vi "metron tester.vi"() -> ()   [LabVIEW 2024]
uses:
  <vilib>/addons/_JKI.lib/REST Client/classes/REST Client/HTTP Header.ctl
  <vilib>/NI/Advanced HTTP Client/Header--Combo Box.ctl
  <vilib>/addons/_JKI.lib/REST Client/classes/REST Client/REST Client.lvclass
  <vilib>/addons/_JKI.lib/Serialization/JSON/JKI JSON Serialization.lvlib
  <vilib>/NI/Advanced HTTP Client/Session.lvclass
panel:
  out "substring":string
  out "Status String":string
  out "text":string
  out "size(s)":i32
  out "Numeric":i32
  out "results":T1(array[cluster])
  out "resulting string":string
  out "Response body":string
  in  "error in (no error)":errorcluster
  out "error out":errorcluster
  in  "resource":string
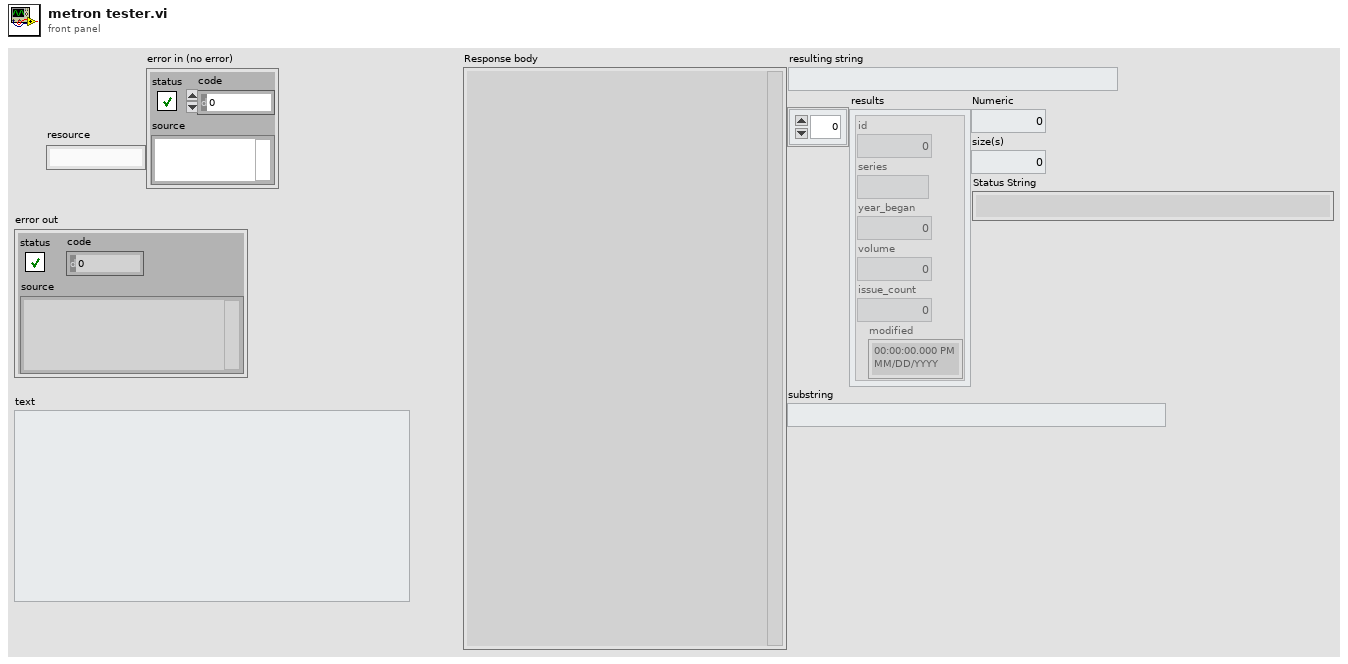
[diagram p1: front panel]
types:
  T1 = cluster{"id":i32, "series":string, "year_began":i32, "volume":i32, "issue_count":i32, "modified":timestamp}[]
  T2 = typedef "REST Client.lvlib/REST Client.lvclass/HTTP Header.ctl" = cluster{"header":T3, "value":string}
  T3 = typedef "lib_NI_Advanced HTTP Client.lvlib/Session.lvclass/Header--Combo Box.ctl" = string
  T4 = cluster{"count":i32, "next":string, "previous":string, "results":cluster{"id":i32, "series":string, "year_began":i32, "volume":i32, "issue_count":i32, "modified":timestamp}[]}
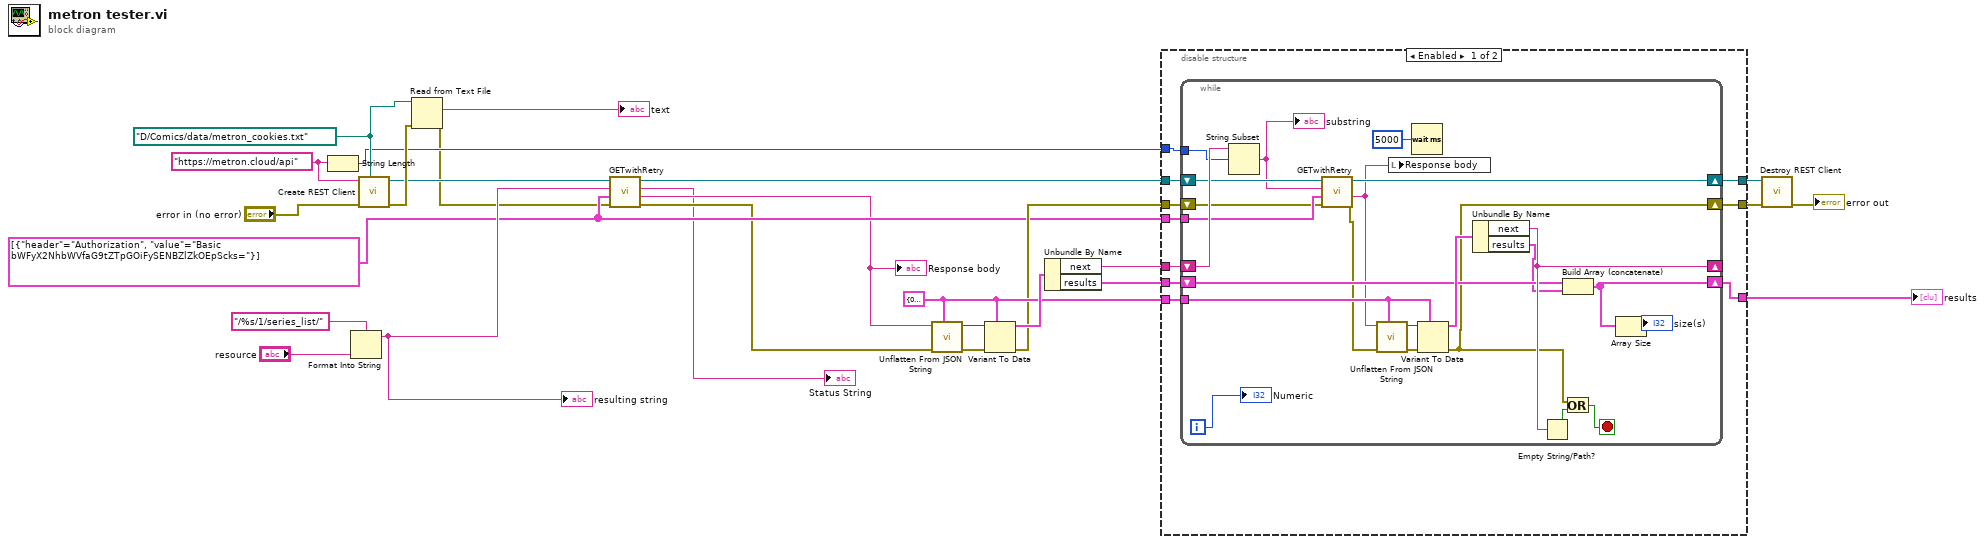
[diagram p0: block diagram]
diagram:
  w5 = T2[] [{"header"="Authorization", "value"="Basic bWFyX2NhbWVfaG9tZTpGOiFySENBZlZkOEpScks="}] ("request specific headers")
  w13 = path "D:/Comics/data/metron_cookies.txt" ("Cookie File")
  w18 = T4 {"count"=0, "next"="", "previous"="", "results"=[]} ("return")
  w11 = "https://metron.cloud/api" ("Base URL")
  n1 = String Length(string=w11) -> (length=w9:i32)
  n2 = Format Into String(format string="/%s/1/series_list/", "resource") -> (resulting string=w6:string)  [unwired: 2 in, 1 out]
  "resulting string" <- w6
  n3 = call <vilib>:"Create REST Client.vi"("Cookie File"=w13, "error in (no error)"="error in (no error)", "Base URL"=w11) -> ("error out"=w14:errorcluster, "REST Client out"=w8:refnum<class "REST Client.lvclass">)  [unwired: 7 in]
  n4 = Read from Text File(file (use dialog)=w13, error in=w14) -> (text=→"text":string, error out=w4:errorcluster)  [unwired: 2 in, 2 out]
  n5 = call "GETwithRetry.vi"("error in (no error)"=w4, "request specific headers"=w5, "String"=w6, "REST Client in"=w8) -> ("error out"=w3:errorcluster, "Response body"=w2:string, "Status String"=→"Status String":string, "REST Client out"=w7:refnum<class "REST Client.lvclass">)  [unwired: 4 in]
  "Response body" <- w2
  n6 = call <vilib>:"Unflatten From JSON String.vi"("Type and Defaults"=w18, "error in (no error)"=w3, "JSON String"=w2) -> ("error out"=w24:errorcluster, "Variant"=w23:variant)  [unwired: 7 in]
  n7 = Variant To Data(error in=w24, type=w18, Variant=w23) -> (data=w22:T4, error out=w16:errorcluster)
  n8 = Unbundle By Name(w22) -> ("next"=w10:string, "results"=w17:T1)
  n9 = disable-structure shown="Enabled" {
    disable-tunnel: w7 -> [w37 w63]
    disable-tunnel: [w36 w63] -> w20
    disable-tunnel: [w35 w62] -> w19
    disable-tunnel: w10 -> [w34 _]
    disable-tunnel: w18 -> [w33 _]
    disable-tunnel: w17 -> [w32 w61]
    disable-tunnel: w16 -> [w31 w62]
    disable-tunnel: [w30 w61] -> w15
    disable-tunnel: w5 -> [w29 _]
    disable-tunnel: w9 -> [w28 _]
    frame Enabled {
      n10 = while {
        shift-right: [w42] -> w36
        shift-left: w37 -> [w43]
        shift-right: [w51] -> w35
        shift-left: w31 -> [w40]
        shift-right: [w56] -> _
        shift-left: w34 -> [w46]
        tunnel: w33 -> [w59]
        shift-right: [w47] -> w30
        shift-left: w32 -> [w55]
        tunnel: w29 -> [w44]
        tunnel: w28 -> [w45]
        i -> [w53]
        stop <- w50 stop-if-true
        n11 = String Subset(string=w46, offset (0)=w45) -> (substring=w39:string)  [unwired: 1 in]
        "substring" <- w39
        n12 = call "GETwithRetry.vi"("error in (no error)"=w40, "request specific headers"=w44, "String"=w39, "REST Client in"=w43) -> ("error out"=w41:errorcluster, "Response body"=w38:string, "REST Client out"=w42:refnum<class "REST Client.lvclass">)  [unwired: 4 in, 1 out]
        n13 = call <vilib>:"Unflatten From JSON String.vi"("Type and Defaults"=w59, "error in (no error)"=w41, "JSON String"=w38) -> ("error out"=w60:errorcluster, "Variant"=w58:variant)  [unwired: 7 in]
        n14 = local write "Response body"(w38) -> ()
        n15 = Wait (ms)(milliseconds to wait=u32 5000) -> ()  [unwired: 1 out]
        n16 = Variant To Data(error in=w60, type=w59, Variant=w58) -> (data=w57:T4, error out=w51:errorcluster)
        n17 = Unbundle By Name(w57) -> ("next"=w56:string, "results"=w54:T1)
        n18 = Empty String/Path?(string/path=w56) -> (empty?=w52:bool)
        n19 = Build Array (concatenate)(w55, w54) -> (w47:T1)
        n20 = Or(x=w51, y=w52) -> (x .or. y?=w50:bool)
        n21 = Array Size(array=w47) -> (size(s)=→"size(s)":i32)
        "Numeric" <- w53
      }
    }
    frame Disabled {
    }
  }
  "results" <- w15
  n22 = call-dynamic "Destroy REST Client.vi"("error in (no error)"=w19, "REST Client in"=w20) -> ("error out"=→"error out":errorcluster)  [unwired: 9 in]
